vi "NSES2_Main.vi"() -> ()   [LabVIEW 2016]
uses:
  Type-Defs/Workspace.ctl
  litho folder/Global/Lithography Data.vi
panel:
  out "Workspace":T1
  in  "s_Path":path=path "C:/Users/monke/Desktop" caption="Path"
  in  "b_lithography_Monitor":bool caption="Blank"
  in  "DAQ Channel":tag
  out "Scan":picture
  out "s_InkScape_path":string="C:\\Users\\monke\\Desktop\\5.8.2018\\5.8.2018\\InkscapeFiles\\5.8.2018.000000.svg" caption="String"
  in  "b_Open_Lithography":bool caption="Config"
  in  "b_Start_Lithography":bool caption="Start"
  in  "b_Change_litho":bool caption="Change"
  in  "l_Litho_modes":i32(ring)=1 caption="Tip Signal Mode" items=["Current Measurement ", "Voltage Source", "Direct from BNC"]
  in  "b_retry_access":bool caption="Reset"
  in  "b_Lithography_Mode":bool caption="Blank"
  in  "b_Open_InkScape":bool caption="Open"
  in  "b_Save_Scan":bool caption="Save"
  in  "b_Config":bool caption="Config"
  # "InkScape should open momentarily.\nHowever, if it fails to load in a reasonable amount of time, below is the path of the InkScape file if needed:"
  # "It appears that you have not \"viewed\" the Access Codes. Please \"view\" them and then press \"RESET\"."
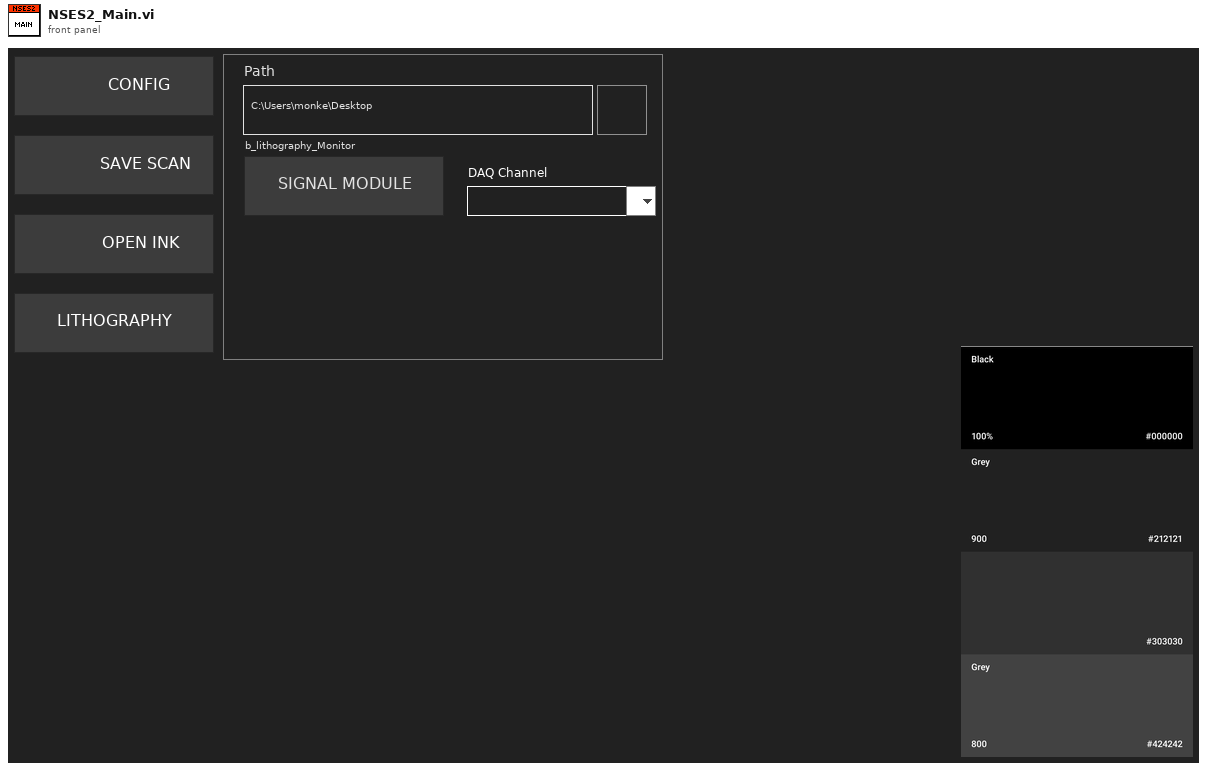
[diagram p1: front panel]
types:
  T1 = typedef "Workspace.ctl" = enum32{"CONFIG", "SAVE SCAN", "OPEN INKSCAPE", "LITHOMODE", "ERROR 97", "MONITOR_LITHO"}
  T2 = enum32{"invalid app kind", "Development System", "Run Time System", "Student Edition", "Embedded LabVIEW", "Evaluation", "Custom"}
  T3 = enum32{"Invalid", "Standard", "Closed", "Hidden", "Minimized", "Maximized"}
  T4 = cluster{"Core":cluster{"Current VI Reference":refnum<vi>, "Close Panel on Exit?":bool}, "lithography_monitor":bool, "Your string data":string, "Main_Path":path, "Image_Paths":cluster{"BMP":string, "BMP_Inkscape":string, "SVG_Inkscape":string}, "Application":refnum<k7>, "lithography_Offsets":cluster{"X":dbl, "Y":dbl}, "Lithography Data":cluster{"Name":string, "Litho":cluster{"X":dbl, "Y":dbl, "Speed":dbl, "Voltage":dbl}[]}[]}
  T5 = cluster{"Name":string, "Litho":cluster{"X":dbl, "Y":dbl, "Speed":dbl, "Voltage":dbl}[]}[]
  T6 = cluster{"BMP":string, "BMP_Inkscape":string, "SVG_Inkscape":string}
  T7 = cluster{"Current VI Reference":refnum<vi>, "Close Panel on Exit?":bool}
  T8 = enum8{"Enabled", "Disabled", "Disabled and Grayed Out"}
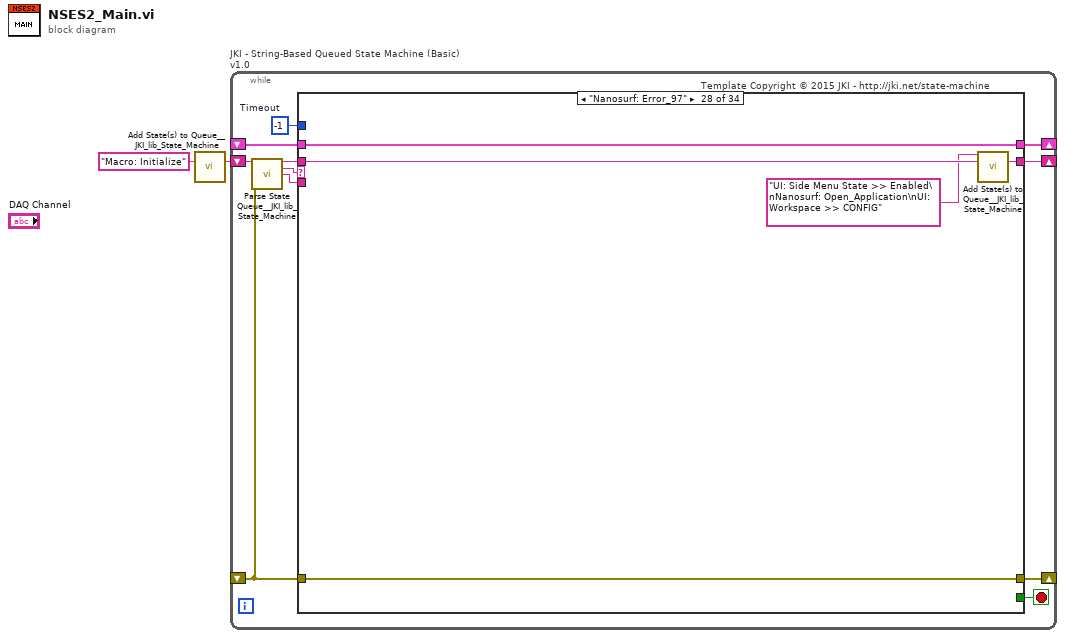
[diagram p0: block diagram]
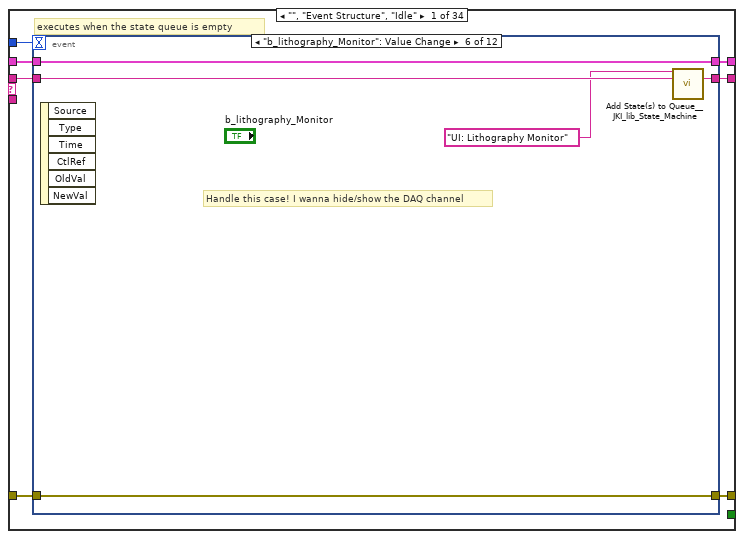
[diagram p2: hidden frame]
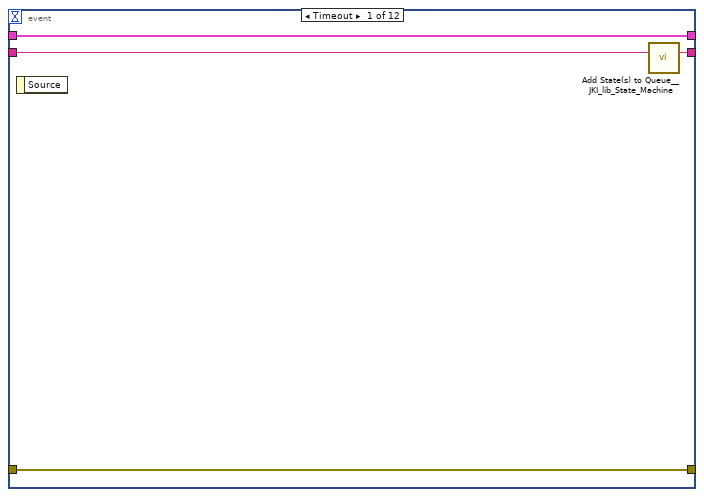
[diagram p3: hidden frame]
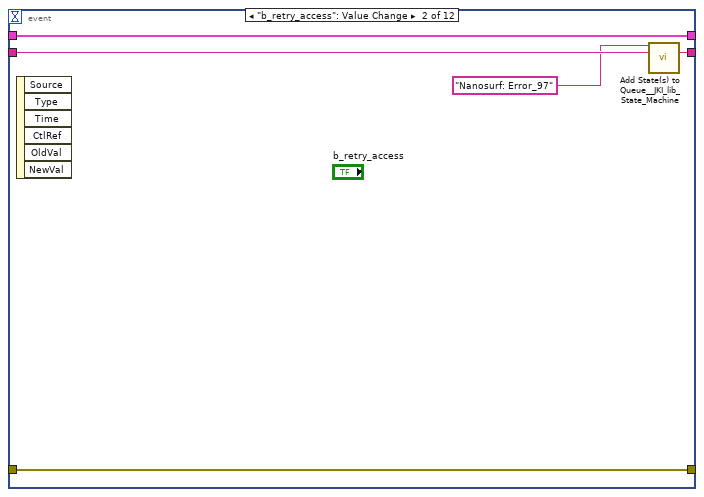
[diagram p4: hidden frame]
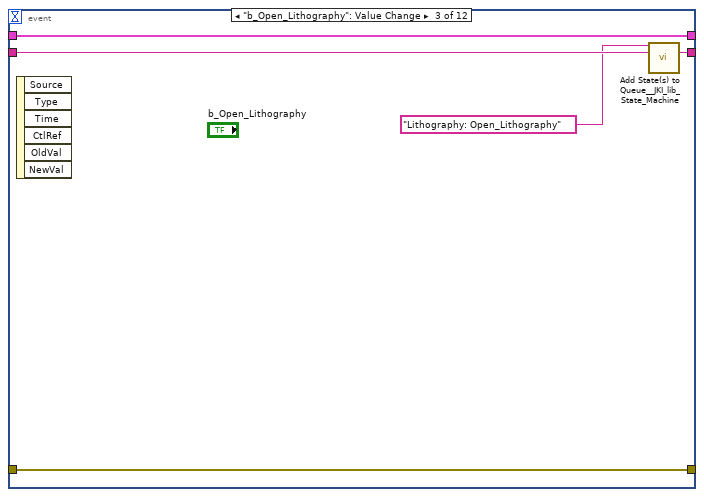
[diagram p5: hidden frame]
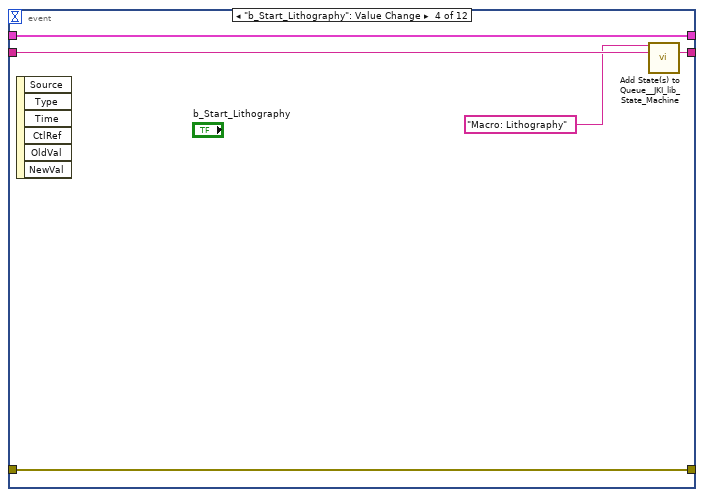
[diagram p6: hidden frame]
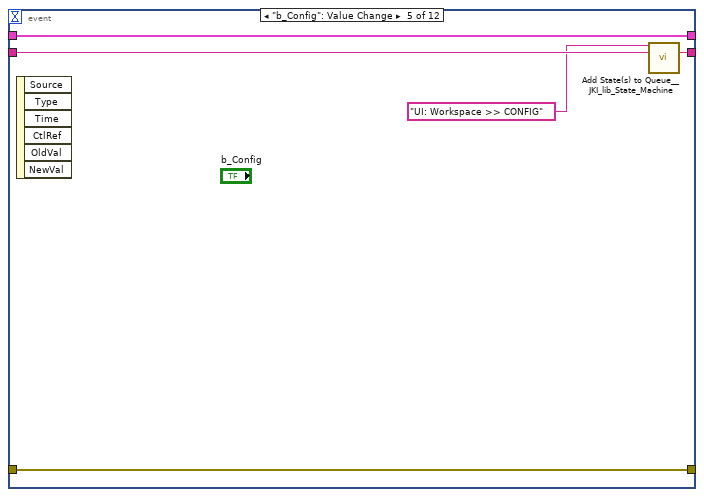
[diagram p7: hidden frame]
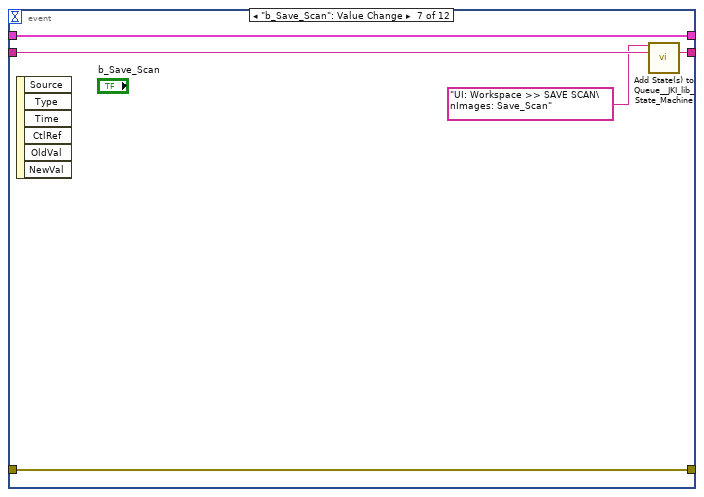
[diagram p8: hidden frame]
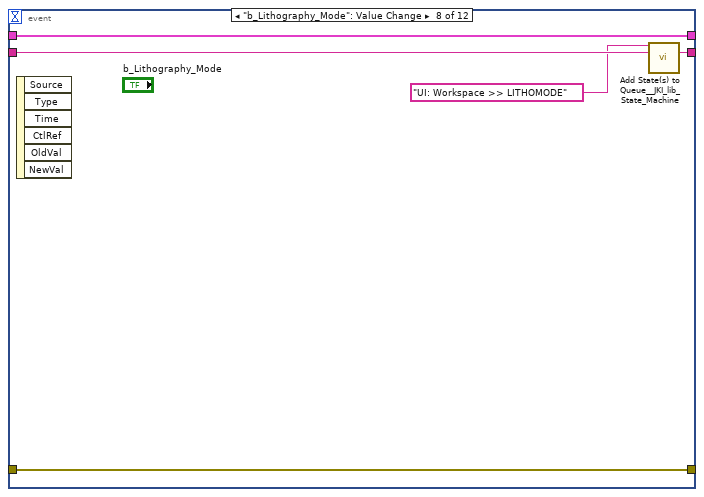
[diagram p9: hidden frame]
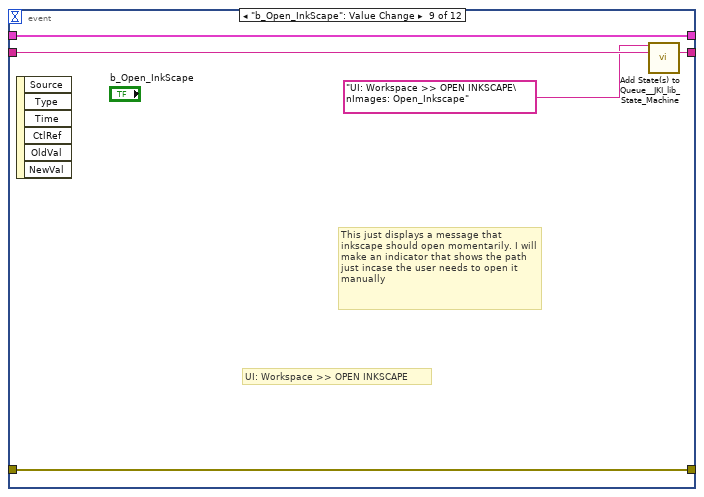
[diagram p10: hidden frame]
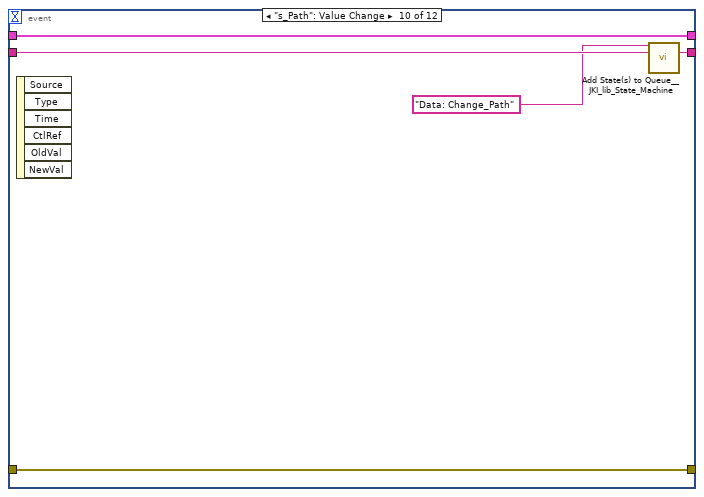
[diagram p11: hidden frame]
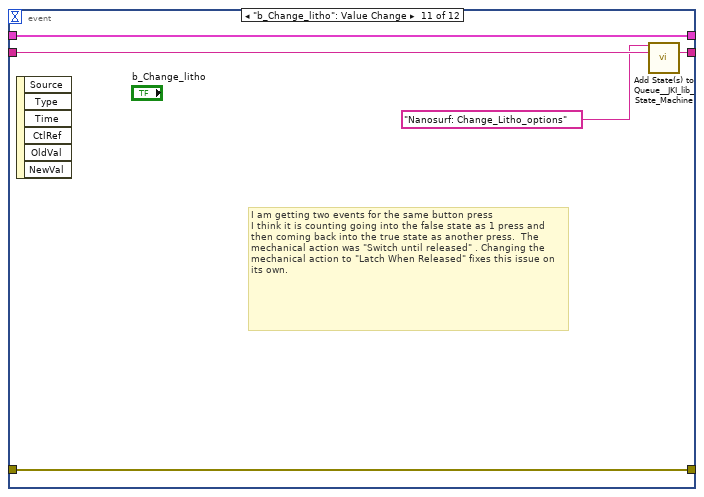
[diagram p12: hidden frame]
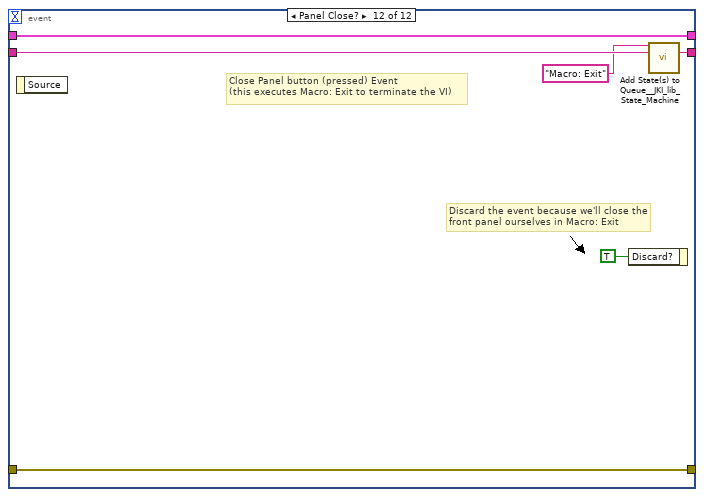
[diagram p13: hidden frame]
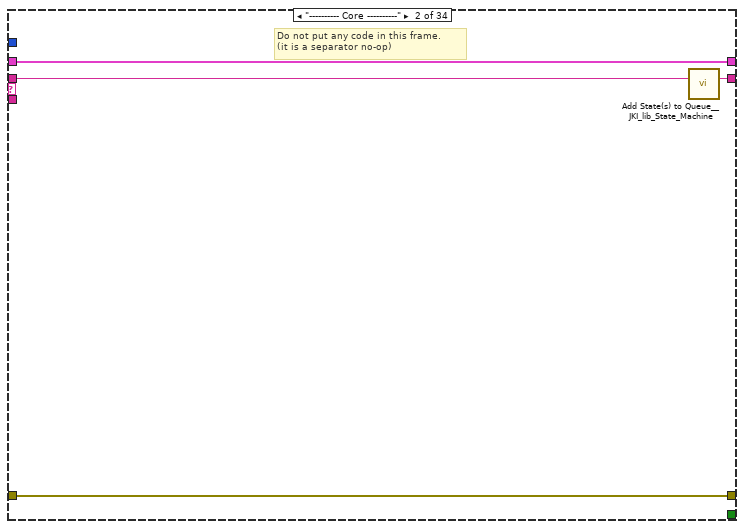
[diagram p14: hidden frame]
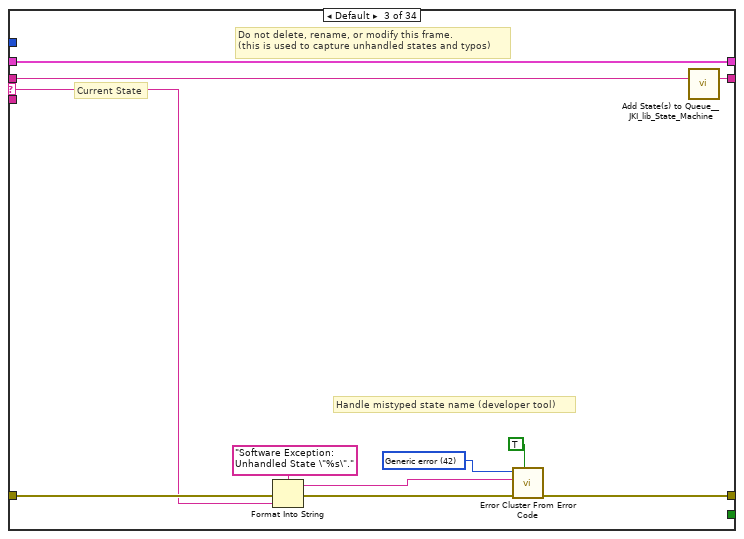
[diagram p15: hidden frame]
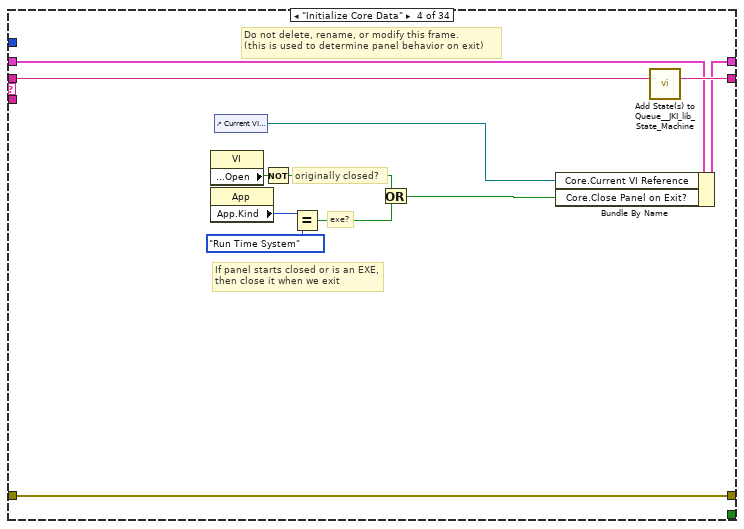
[diagram p16: hidden frame]
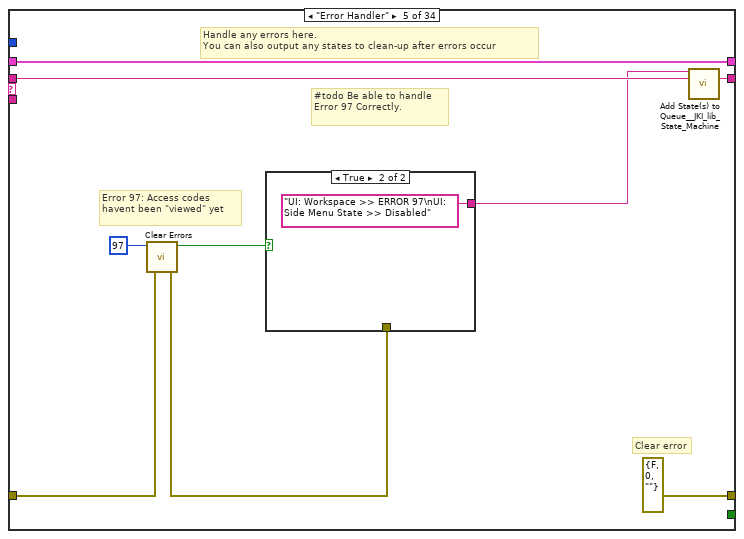
[diagram p17: hidden frame]
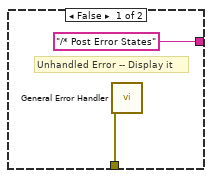
[diagram p18: hidden frame]
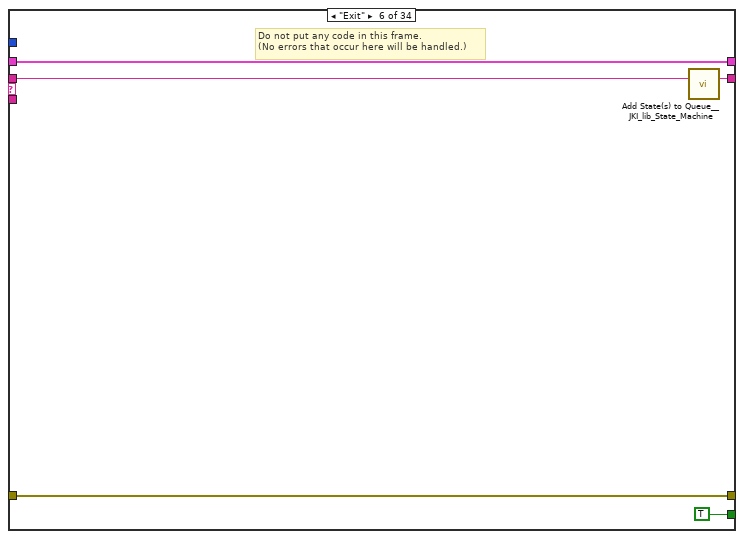
[diagram p19: hidden frame]
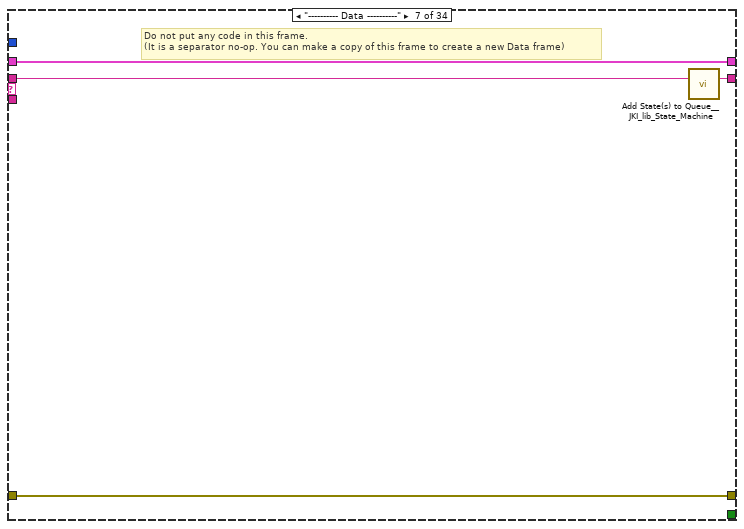
[diagram p20: hidden frame]
diagram:
  n1 = call <vilib>:"Add State(s) to Queue__JKI_lib_State_Machine.vi"("State(s) in (\"\")"="Macro: Initialize") -> ("States Out"=w2:string)  [unwired: 14 in]
  n2 = while "JKI - String-Based Queued State Machine (Basic) v1.0" {
    shift-right: [w7] -> _
    shift-left: _ -> [w6]
    shift-right: [w9] -> _
    shift-left: _ -> [w4]
    shift-right: [w3] -> _
    shift-left: w2 -> [w10]
    stop <- w8 stop-if-true
    w5 = -1  # Timeout
    # "Template Copyright © 2015 JKI - http://jki.net/state-machine"
    n3 = call <vilib>:"Parse State Queue__JKI_lib_State_Machine.vi"("State Queue"=w10, "Error In (no error)"=w4) -> ("Remaining States"=w12:string, "Current State"=w13:string, "Arguments"=w11:string)  [unwired: 11 in]
    n4 = case shown="\"Nanosurf: Error_97\"" w13 {
      selector: w13 -> [_ _ w85 _ _ _ _ _ _ _ _ _ _ _ _ _ _ _ _ _ _ _ _ _ _ _ _ _ _ _ _ _ _ _]
      tunnel: w12 -> [w20 w84 w89 w107 w116 w124 w128 w140 w146 w152 w156 w160 w166 w177 w205 w216 w234 w238 w243 w255 w265 w269 w282 w293 w297 w305 w312 w317 w323 w327 w338 w350 w359 w364]
      tunnel: w11 -> [_ _ _ _ _ _ _ _ _ _ _ _ w161 w171 w201 w211 _ _ _ _ _ _ _ _ _ _ _ _ _ _ _ _ _ w360]
      tunnel: w6 -> [w18 w81 w87 w98 w113 w122 w125 _ w143 w147 w153 w158 w164 w173 w202 w214 w230 w235 w240 w249 w262 w267 w275 w284 w294 w299 w310 w315 w319 w324 w329 w346 w355 w361]
      tunnel: [w17 w82 w91 w104 errorcluster {"status"=FALSE, "code"=0, "source"=""} ("error out") w121 w126 w137 w144 w148 w154 w157 w162 w174 w203 w212 w232 w236 w241 w253 w263 w266 w278 w285 w295 w301 w306 w313 w320 w325 w330 w340 w356 w362] -> w9
      tunnel: w4 -> [w16 w82 w90 w104 w110 w121 w126 w137 w144 w149 w154 w157 w163 w175 w203 w213 w232 w236 w241 w253 w263 w266 w279 w286 w295 w302 w307 w313 w321 w325 w331 w348 w357 w362]
      tunnel: [w19 w83 w88 w106 w115 w123 w127 w139 w145 w151 w155 w159 w165 w176 w204 w215 w233 w237 w242 w254 w264 w268 w281 w292 w296 w304 w311 w316 w322 w326 w337 w349 w358 w363] -> w3
      tunnel: [_ _ _ _ _ TRUE _ _ _ _ _ _ _ _ _ _ _ _ _ _ _ _ _ _ _ _ _ _ _ _ _ _ _ _] -> w8
      tunnel: [w15 w81 w87 w105 w113 w122 w125 w138 w142 w147 w153 w158 w164 w173 w202 w214 w229 w235 w240 w249 w262 w267 w274 w284 w294 w298 w310 w315 w319 w324 w329 w345 w355 w361] -> w7
      tunnel: w5 -> [w14 _ _ _ _ _ _ _ _ _ _ _ _ _ _ _ _ _ _ _ _ _ _ _ _ _ _ _ _ _ _ _ _ _]
      frame "", "Event Structure", "Idle" {
        # "executes when the state queue is empty"
        n5 = event shown="[5] \"b_lithography_Monitor\": Value Change" {
          selector: _ -> [_ _ _ _ _ _ _ _ _ _ _ _]
          dyn-events: _ -> [_ _ _ _ _ _ _ _ _ _ _ _]
          timeout: w14 -> [_ _ _ _ _ _ _ _ _ _ _ _]
          tunnel: w20 -> [w24 w29 w34 w39 w44 w49 w54 w59 w64 w69 w74 w80]
          tunnel: [w23 w28 w33 w38 w43 w48 w53 w58 w63 w68 w73 w79] -> w19
          tunnel: w18 -> [w21 w26 w31 w36 w41 w46 w51 w56 w61 w66 w71 w77]
          tunnel: [w22 w27 w32 w37 w42 w47 w52 w57 w62 w67 w72 w78] -> w17
          tunnel: w16 -> [w22 w27 w32 w37 w42 w47 w52 w57 w62 w67 w72 w78]
          tunnel: [w21 w26 w31 w36 w41 w46 w51 w56 w61 w66 w71 w77] -> w15
          event Timeout {
            n6 = event-data() -> ()  [unwired: 1 in, 1 out]
            n7 = call <vilib>:"Add State(s) to Queue__JKI_lib_State_Machine.vi"("State(s) in (\"\")"=w24) -> ("States Out"=w23:string)  [unwired: 14 in]
          }
          event "b_retry_access": Value Change {
            n8 = event-data() -> ()  [unwired: 1 in, 6 out]
            n9 = call <vilib>:"Add State(s) to Queue__JKI_lib_State_Machine.vi"("State(s) in Front (\"\")"="Nanosurf: Error_97" ("State(s) in Front (\"\")"), "State(s) in (\"\")"=w29) -> ("States Out"=w28:string)  [unwired: 13 in]
          }
          event "b_Open_Lithography": Value Change {
            n10 = event-data() -> ()  [unwired: 1 in, 6 out]
            n11 = call <vilib>:"Add State(s) to Queue__JKI_lib_State_Machine.vi"("State(s) in Front (\"\")"="Lithography: Open_Lithography" ("State(s) in Front (\"\")"), "State(s) in (\"\")"=w34) -> ("States Out"=w33:string)  [unwired: 13 in]
          }
          event "b_Start_Lithography": Value Change {
            n12 = event-data() -> ()  [unwired: 1 in, 6 out]
            n13 = call <vilib>:"Add State(s) to Queue__JKI_lib_State_Machine.vi"("State(s) in Front (\"\")"="Macro: Lithography" ("State(s) in Front (\"\")"), "State(s) in (\"\")"=w39) -> ("States Out"=w38:string)  [unwired: 13 in]
          }
          event "b_Config": Value Change {
            n14 = event-data() -> ()  [unwired: 1 in, 6 out]
            n15 = call <vilib>:"Add State(s) to Queue__JKI_lib_State_Machine.vi"("State(s) in Front (\"\")"="UI: Workspace >> CONFIG" ("State(s) in Front (\"\")"), "State(s) in (\"\")"=w44) -> ("States Out"=w43:string)  [unwired: 13 in]
          }
          event "b_lithography_Monitor": Value Change {
            # "Handle this case! I wanna hide/show the DAQ channel"
            n16 = event-data() -> ()  [unwired: 1 in, 6 out]
            n17 = call <vilib>:"Add State(s) to Queue__JKI_lib_State_Machine.vi"("State(s) in Front (\"\")"="UI: Lithography Monitor" ("State(s) in Front (\"\")"), "State(s) in (\"\")"=w49) -> ("States Out"=w48:string)  [unwired: 13 in]
          }
          event "b_Save_Scan": Value Change {
            n18 = event-data() -> ()  [unwired: 1 in, 6 out]
            n19 = call <vilib>:"Add State(s) to Queue__JKI_lib_State_Machine.vi"("State(s) in Front (\"\")"="UI: Workspace >> SAVE SCAN\nImages: Save_Scan" ("State(s) in Front (\"\")"), "State(s) in (\"\")"=w54) -> ("States Out"=w53:string)  [unwired: 13 in]
          }
          event "b_Lithography_Mode": Value Change {
            n20 = event-data() -> ()  [unwired: 1 in, 6 out]
            n21 = call <vilib>:"Add State(s) to Queue__JKI_lib_State_Machine.vi"("State(s) in Front (\"\")"="UI: Workspace >> LITHOMODE" ("State(s) in Front (\"\")"), "State(s) in (\"\")"=w59) -> ("States Out"=w58:string)  [unwired: 13 in]
          }
          event "b_Open_InkScape": Value Change {
            # "This just displays a message that inkscape should open momentarily. I will make an indicator that shows the path just incase the user needs to open it manually"
            # "UI: Workspace >> OPEN INKSCAPE"
            n22 = event-data() -> ()  [unwired: 1 in, 6 out]
            n23 = call <vilib>:"Add State(s) to Queue__JKI_lib_State_Machine.vi"("State(s) in Front (\"\")"="UI: Workspace >> OPEN INKSCAPE\nImages: Open_Inkscape" ("State(s) in Front (\"\")"), "State(s) in (\"\")"=w64) -> ("States Out"=w63:string)  [unwired: 13 in]
          }
          event "s_Path": Value Change {
            n24 = event-data() -> ()  [unwired: 1 in, 6 out]
            n25 = call <vilib>:"Add State(s) to Queue__JKI_lib_State_Machine.vi"("State(s) in Front (\"\")"="Data: Change_Path" ("State(s) in Front (\"\")"), "State(s) in (\"\")"=w69) -> ("States Out"=w68:string)  [unwired: 13 in]
          }
          event "b_Change_litho": Value Change {
            # "I am getting two events for the same button press \nI think it is counting going into the false state as 1 press and then coming back into the true state as another press.  The mechanical action was \"Switch until released\" . Changing the mechanical action to \"Latch When Released\" fixes this issue on its own."
            n26 = event-data() -> ()  [unwired: 1 in, 6 out]
            n27 = call <vilib>:"Add State(s) to Queue__JKI_lib_State_Machine.vi"("State(s) in Front (\"\")"="Nanosurf: Change_Litho_options", "State(s) in (\"\")"=w74) -> ("States Out"=w73:string)  [unwired: 13 in]
          }
          event Panel Close? {
            # "Discard the event because we'll close the front panel ourselves in Macro: Exit"
            # "Close Panel button (pressed) Event\n(this executes Macro: Exit to terminate the VI)"
            n28 = event-data() -> ()  [unwired: 1 in, 1 out]
            n29 = event-data("Discard?"=TRUE) -> ()  [unwired: 1 in, 1 out]
            n30 = call <vilib>:"Add State(s) to Queue__JKI_lib_State_Machine.vi"("State(s) in Front (\"\")"="Macro: Exit", "State(s) in (\"\")"=w80) -> ("States Out"=w79:string)  [unwired: 13 in]
          }
        }
      }
      frame "---------- Core ----------" {
        # "Do not put any code in this frame.\n(it is a separator no-op)"
        n31 = call <vilib>:"Add State(s) to Queue__JKI_lib_State_Machine.vi"("State(s) in (\"\")"=w84) -> ("States Out"=w83:string)  [unwired: 14 in]
      }
      frame Default {
        w94 = 42 items=["No error", "Argument error", "Memory is full", "Out of zone", "End of file", "File already open", "Generic file I/O error", "File not found", "File permission error", "Disk is full", "Duplicate path", "Too many files open", "System feature not enabled", "Resource file not found", "Cannot add resource", "Resource not found", "Image not found", "Image memory error", "Pen does not exist", "Config type invalid", "Config token not found", "Config parse error", "Config memory error", "Bad external code format", "Bad external code offset", "External code not present", "Null window", "Destroy window error", "Null menu", "Print aborted", "Bad print record", "Print driver error", "Windows error during printing", "Memory error during printing", "Print dialog error", "Generic print error", "Invalid device refnum", "Device not found", "Device parameter error", "Device unit error", "Cannot open device", "Device call aborted", "Generic error", "Cancelled by user", "Object ID too low", "Object ID too high", "Object not in heap", "Unknown heap", "Unknown object (invalid DefProc)", "Unknown object (DefProc not in table)", "Message out of range", "Invalid (null) method", "Unknown message", "Manager call not supported", "Bad address", "Network operation in progress", "Network operation timed out", "Connection is busy", "Network attribute not supported", "Network error", "Address in use", "System out of memory", "Connection aborted", "Connection refused", "Not connected", "Already connected", "Connection closed", "Initialization error (interapplication manager)", "Bad occurrence", "Wait on unbound occurrence handler", "Occurrence queue overflow", "Datalog type conflict", "Unused", "Unrecognized type (interapplication manager)", "Memory corrupt", "Failed to make temporary DLL", "Old CIN version", "Drag socket not found", "Failed to load drop-object", "Failed to register OLE object", "Failed to release OLE object", "Format specifier type mismatch", "Unknown format specifier", "Too few format specifiers", "Too many format specifiers", "Scan failed", "Newer CIN version", "Error converting to variant", "Runtime menu error", "Password tampered", "Variant attribute not found", "Incompatible variant data type", "Event data is not available", "Event Store is not present", "Occurrence is not found", "Event Queue is not created", "Event info is not available", "Refnum passed is NULL", "Error retrieving Class GUID", "Error retrieving CoClass GUID", "Error retrieving TypeLib GUID.", "Bad built application magic bytes.", "Specific driver is different from the specific driver associated with the Logical Name.", "There is no session opened to the class driver.", "Max Error", "MAX - Error with config objects", "MAX - Error loading configuration", "MAX - Group not supported"]
        # "Current State"
        # "Do not delete, rename, or modify this frame.\n(this is used to capture unhandled states and typos)"
        # "Handle mistyped state name (developer tool)"
        n32 = Format Into String(format string="Software Exception: Unhandled State \"%s\"." ("message"), error in=w90, w85) -> (resulting string=w93:string, error out=w92:errorcluster)  [unwired: 1 in]
        n33 = call <vilib>:"Error Cluster From Error Code.vi"("show call chain? (False)"=TRUE, "error in (no error)"=w92, "error message (\"\")"=w93, "error code (0)"=w94) -> ("error out"=w91:errorcluster)  [unwired: 5 in]
        n34 = call <vilib>:"Add State(s) to Queue__JKI_lib_State_Machine.vi"("State(s) in (\"\")"=w89) -> ("States Out"=w88:string)  [unwired: 14 in]
      }
      frame "Initialize Core Data" {
        # "Do not delete, rename, or modify this frame.\n(this is used to determine panel behavior on exit)"
        # "originally closed?"
        # "exe?"
        # "If panel starts closed or is an EXE, then close it when we exit"
        n35 = property class="VI"() -> ("Front Panel.Open"=w103:bool)  [unwired: 2 in, 2 out]
        n36 = property class="App"() -> ("App.Kind"=w102:T2)  [unwired: 2 in, 2 out]
        n37 = control-ref of="Current VI Reference"() -> (w96:refnum<vi>)
        n38 = Not(x=w103) -> (.not. x?=w100:bool)
        n39 = Equal?(x=w102, y=T2."Run Time System" ("Application:Kind")) -> (x = y?=w99:bool)
        n40 = Or(x=w100, y=w99) -> (x .or. y?=w97:bool)
        n41 = Bundle By Name(cluster=w98, "Core.Current VI Reference"=w96, "Core.Close Panel on Exit?"=w97) -> (w105:T4)
        n42 = call <vilib>:"Add State(s) to Queue__JKI_lib_State_Machine.vi"("State(s) in (\"\")"=w107) -> ("States Out"=w106:string)  [unwired: 14 in]
      }
      frame "Error Handler" {
        # "Error 97: Access codes havent been \"viewed\" yet"
        # "#todo Be able to handle Error 97 Correctly."
        # "Handle any errors here.\nYou can also output any states to clean-up after errors occur"
        # "Clear error"
        n43 = call <vilib>:"Clear Errors.vi"("error in (no error)"=w110, "specific error code to clear (0: all)"=97) -> ("error out"=w109:errorcluster, "specific error cleared?"=w111:bool)  [unwired: 4 in]
        n44 = case shown="True" w111 {
          tunnel: w109 -> [w118 _]
          tunnel: ["/* Post Error States" "UI: Workspace >> ERROR 97\nUI: Side Menu State >> Disabled"] -> w108
          frame False {
            # "Unhandled Error -- Display it"
            n45 = call <vilib>:"General Error Handler.vi"("error in (no error)"=w118) -> ()  [unwired: 10 in, 5 out]
          }
          frame True {
          }
        }
        n46 = call <vilib>:"Add State(s) to Queue__JKI_lib_State_Machine.vi"("State(s) in Front (\"\")"=w108, "State(s) in (\"\")"=w116) -> ("States Out"=w115:string)  [unwired: 13 in]
      }
      frame "Exit" {
        # "Do not put any code in this frame.\n(No errors that occur here will be handled.)"
        n47 = call <vilib>:"Add State(s) to Queue__JKI_lib_State_Machine.vi"("State(s) in (\"\")"=w124) -> ("States Out"=w123:string)  [unwired: 14 in]
      }
      frame "---------- Data ----------" {
        # "Do not put any code in this frame.\n(It is a separator no-op. You can make a copy of this frame to create a new Data frame)"
        n48 = call <vilib>:"Add State(s) to Queue__JKI_lib_State_Machine.vi"("State(s) in (\"\")"=w128) -> ("States Out"=w127:string)  [unwired: 14 in]
      }
      frame "Data: Initialize" {
        w129 = T5 []  # Lithography Data
        w130 = cluster{"X":dbl, "Y":dbl} {"X"=0.0, "Y"=0.0}  # lithography_Offsets
        w131 = refnum<k7> refnum  # Application
        w132 = T6 {"BMP"="", "BMP_Inkscape"="", "SVG_Inkscape"=""}  # Image_Paths
        w133 = path ""  # Main_Path
        w134 = T7 {"Current VI Reference"=refnum, "Close Panel on Exit?"=FALSE}  # Core
        w136 = TRUE  # lithography_monitor
        w135 = ""  # Your string data
        # "Initialize the shift-register data, here.\n(data names are defined by what you wire into the bundle function)"
        n49 = Bundle("Core"=w134, "lithography_monitor"=w136, "Your string data"=w135, "Main_Path"=w133, "Image_Paths"=w132, "Application"=w131, "lithography_Offsets"=w130, "Lithography Data"=w129) -> (w138:T4)  [unwired: 1 in]
        n50 = call <vilib>:"Add State(s) to Queue__JKI_lib_State_Machine.vi"("State(s) in (\"\")"=w140) -> ("States Out"=w139:string)  [unwired: 14 in]
      }
      frame "Data: Change_Path" {
        # "Do not put any code in this frame.\n(It is a separator no-op. You can make a copy of this frame to create a new Data frame)"
        n51 = Bundle By Name(cluster=w143, "Main_Path"="s_Path") -> (w142:T4)
        n52 = call <vilib>:"Add State(s) to Queue__JKI_lib_State_Machine.vi"("State(s) in (\"\")"=w146) -> ("States Out"=w145:string)  [unwired: 14 in]
      }
      frame "Data: Cleanup" {
        # "Cleanup any data and references, here.\n(this is called automatically, by the Macro: Exit)"
        n53 = Unbundle By Name(w147) -> ("Core.Current VI Reference"=w150:refnum<vi>)
        n54 = Close Reference(reference=w150, error in (no error)=w149) -> (error out=w148:errorcluster)
        n55 = call <vilib>:"Add State(s) to Queue__JKI_lib_State_Machine.vi"("State(s) in (\"\")"=w152) -> ("States Out"=w151:string)  [unwired: 14 in]
      }
      frame "---------- UI ----------" {
        # "Do not put any code in this frame.\n(It is a separator no-op. You can make a copy of this frame to create a new UI frame)"
        n56 = call <vilib>:"Add State(s) to Queue__JKI_lib_State_Machine.vi"("State(s) in (\"\")"=w156) -> ("States Out"=w155:string)  [unwired: 14 in]
      }
      frame "UI: Initialize" {
        # "Initialize the User Interface, here.\n(this is called automatically, by the Macro: Init)"
        n57 = call <vilib>:"Add State(s) to Queue__JKI_lib_State_Machine.vi"("State(s) in (\"\")"=w160) -> ("States Out"=w159:string)  [unwired: 14 in]
      }
      frame "UI: Cursor Set" {
        # "Argument"
        # "Set and Unset Cursor Busy.\n(Usage: \"UI: Cursor Set >> Busy|Idle\")"
        n58 = case shown="\"Idle\", Default" w161 {
          tunnel: w163 -> [w168 w170]
          tunnel: [w167 w169] -> w162
          frame "Idle", Default {
            n59 = call <vilib>:"Unset Busy.vi"("error in (no error)"=w168) -> ("error out"=w167:errorcluster)  [unwired: 10 in]
          }
          frame "Busy" {
            n60 = call <vilib>:"Set Busy.vi"("error in (no error)"=w170) -> ("error out"=w169:errorcluster)  [unwired: 9 in, 1 out]
          }
        }
        n61 = call <vilib>:"Add State(s) to Queue__JKI_lib_State_Machine.vi"("State(s) in (\"\")"=w166) -> ("States Out"=w165:string)  [unwired: 14 in]
      }
      frame "UI: Front Panel State" {
        # "Argument"
        # "Set Front Panel Open or Closed\n(Usage: \"UI: Front Panel State >> Open|Close\")"
        n62 = Unbundle By Name(w173) -> ("Core.Current VI Reference"=w172:refnum<vi>)
        n63 = case shown="\"Open\", Default" w171 {
          tunnel: w175 -> [w181 w194]
          tunnel: [w183 w195] -> w174
          tunnel: w172 -> [w182 w192]
          frame "Open", Default {
            n64 = property class="VI"(reference=w182, error in=w181) -> (reference out=w179:refnum<vi>, error out=w180:errorcluster, "Front Panel.Open"=w178:bool)
            n65 = case shown="False" w178 {
              tunnel: [w186 w189] -> w183
              tunnel: w180 -> [w185 w189]
              tunnel: w179 -> [w184 _]
              frame False {
                n66 = invoke class="VI" method="FP.Open"(reference=w184, error in=w185, "Activate"=TRUE, "State"=T3."Standard") -> (error out=w186:errorcluster)  [unwired: 1 in, 4 out]
              }
              frame True {
              }
            }
          }
          frame "Close" {
            n67 = property class="VI"(reference=w192, error in=w194) -> (reference out=w191:refnum<vi>, error out=w193:errorcluster, "Front Panel.Open"=w190:bool)
            n68 = case shown="True" w190 {
              tunnel: [w196 w199] -> w195
              tunnel: w193 -> [w196 w198]
              tunnel: w191 -> [_ w197]
              frame False {
              }
              frame True {
                n69 = invoke class="VI" method="FP.Close"(reference=w197, error in=w198) -> (error out=w199:errorcluster)  [unwired: 1 in, 2 out]
              }
            }
          }
        }
        n70 = call <vilib>:"Add State(s) to Queue__JKI_lib_State_Machine.vi"("State(s) in (\"\")"=w177) -> ("States Out"=w176:string)  [unwired: 14 in]
      }
      frame "UI: Workspace" {
        # "Workspace Tab State\n(This is the frame that changes the Workspace Value)"
        n71 = case shown="\"CONFIG\", Default" w201 {
          tunnel: [Workspace."CONFIG" ("Workspace") Workspace."SAVE SCAN" ("Workspace") Workspace."OPEN INKSCAPE" ("Workspace") Workspace."ERROR 97" ("Workspace") Workspace."LITHOMODE" ("Workspace")] -> w200
          frame "CONFIG", Default {
            # "UI: Workspace >> CONFIG"
          }
          frame "SAVE SCAN" {
            # "UI: Workspace >> SAVE SCAN"
          }
          frame "OPEN INKSCAPE" {
            # "UI: Workspace >> OPEN INKSCAPE"
          }
          frame "ERROR 97" {
            # "UI: Workspace >> ERROR 97"
          }
          frame "LITHOMODE" {
            # "UI: Workspace >> LITHOMODE"
          }
        }
        "Workspace" <- w200
        n72 = call <vilib>:"Add State(s) to Queue__JKI_lib_State_Machine.vi"("State(s) in (\"\")"=w205) -> ("States Out"=w204:string)  [unwired: 14 in]
      }
      frame "UI: Side Menu State" {
        # "Do not put any code in this frame.\n(It is a separator no-op. You can make a copy of this frame to create a new UI frame)"
        n73 = case shown="\"Disabled\"" w211 {
          tunnel: w213 -> [w222 w228]
          tunnel: [w221 w227] -> w212
          frame "Disabled" {
            w217 = T8."Disabled and Grayed Out" ("Disabled")
            n74 = property on="b_Config" class="Bool"(error in=w222, "DisabledEnum"=w217) -> (error out=w218:errorcluster)  [unwired: 1 in, 1 out]
            n75 = property on="b_Save_Scan" class="Bool"(error in=w218, "DisabledEnum"=w217) -> (error out=w219:errorcluster)  [unwired: 1 in, 1 out]
            n76 = property on="b_Open_InkScape" class="Bool"(error in=w219, "DisabledEnum"=w217) -> (error out=w220:errorcluster)  [unwired: 1 in, 1 out]
            n77 = property on="b_Lithography_Mode" class="Bool"(error in=w220, "DisabledEnum"=w217) -> (error out=w221:errorcluster)  [unwired: 1 in, 1 out]
          }
          frame "Enabled", Default {
            w223 = T8."Enabled" ("Disabled")
            n78 = property on="b_Config" class="Bool"(error in=w228, "DisabledEnum"=w223) -> (error out=w224:errorcluster)  [unwired: 1 in, 1 out]
            n79 = property on="b_Save_Scan" class="Bool"(error in=w224, "DisabledEnum"=w223) -> (error out=w225:errorcluster)  [unwired: 1 in, 1 out]
            n80 = property on="b_Open_InkScape" class="Bool"(error in=w225, "DisabledEnum"=w223) -> (error out=w226:errorcluster)  [unwired: 1 in, 1 out]
            n81 = property on="b_Lithography_Mode" class="Bool"(error in=w226, "DisabledEnum"=w223) -> (error out=w227:errorcluster)  [unwired: 1 in, 1 out]
          }
        }
        n82 = call <vilib>:"Add State(s) to Queue__JKI_lib_State_Machine.vi"("State(s) in (\"\")"=w216) -> ("States Out"=w215:string)  [unwired: 14 in]
      }
      frame "UI: Lithography Monitor" {
        # "#b_lithography_Monitor"
        # "Do not put any code in this frame.\n(It is a separator no-op. You can make a copy of this frame to create a new UI frame)"
        n83 = local read "b_lithography_Monitor"() -> (w231:bool)
        n84 = Bundle By Name(cluster=w230, "lithography_monitor"=w231) -> (w229:T4)
        n85 = property on="DAQ Channel" class="DAQName"("Visible"=w231) -> ()  [unwired: 2 in, 2 out]
        n86 = call <vilib>:"Add State(s) to Queue__JKI_lib_State_Machine.vi"("State(s) in (\"\")"=w234) -> ("States Out"=w233:string)  [unwired: 14 in]
      }
      frame "---------- Macro ----------" {
        # "Do not put any code in this frame.\n(It is a separator no-op. You can make a copy of this frame to create a new Macro frame)"
        n87 = call <vilib>:"Add State(s) to Queue__JKI_lib_State_Machine.vi"("State(s) in (\"\")"=w238) -> ("States Out"=w237:string)  [unwired: 14 in]
      }
      frame "Macro: Initialize" {
        w239 = "Data: Initialize\nInitialize Core Data\nUI: Initialize\nUI: Front Panel State >> Open\nUI: Workspace >> CONFIG\nUI: Lithography Monitor\nNanosurf: Open_Application\nData: Change_Path"  # Data: Initialize Initialize Core Data UI: Initialize UI: Front Panel State >> Open UI: Workspace >> CONFIG UI: Lithography Monitor Nanosurf: Open_Application Data: Change_Path
        # "Initialization Macro\n(This is called once, when the VI starts)"
        n88 = call <vilib>:"Add State(s) to Queue__JKI_lib_State_Machine.vi"("State(s) in Front (\"\")"=w239, "State(s) in (\"\")"=w243) -> ("States Out"=w242:string)  [unwired: 13 in]
      }
      frame "Macro: Lithography" {
        # "Do not put any code in this frame.\n(It is a separator no-op. You can make a copy of this frame to create a new Macro frame)"
        n89 = Unbundle By Name(w249) -> ("lithography_monitor"=w248:bool)
        n90 = Select(t="DAQ Card" ("State"), s=w248, f="Signal Module" ("State")) -> (s? t:f=w251:string)
        n91 = call <vilib>:"Build State String with Arguments__JKI_lib_State_Machine.vi"("Arguments (\"\")"=w251, "State"="Lithography: Run") -> ("State with Arguments"=w246:string)  [unwired: 4 in]
        n92 = call <vilib>:"Add State(s) to Queue__JKI_lib_State_Machine.vi"("State(s) in (\"\")"="Lithography: Init\nLithography: Queue", "State(s) at Back (\"\")"=w246) -> ("States Out"=w244:string)  [unwired: 13 in]
        n93 = call <vilib>:"Add State(s) to Queue__JKI_lib_State_Machine.vi"("State(s) in Front (\"\")"=w244, "State(s) in (\"\")"=w255) -> ("States Out"=w254:string)  [unwired: 13 in]
      }
      frame "Macro: Exit" {
        # "Exit Macro\n(This is called once, when the VI exits)"
        n94 = Unbundle By Name(w262) -> ("Core.Close Panel on Exit?"=w261:bool)
        n95 = Select(t="UI: Front Panel State >> Close", s=w261, f="") -> (s? t:f=w258:string)
        n96 = call <vilib>:"Add State(s) to Queue__JKI_lib_State_Machine.vi"("State(s) in (\"\")"=w258, "State(s) at Back (\"\")"="UI: Workspace >> CONFIG\nNanosurf: Close_Application\nData: Cleanup\nExit") -> ("States Out"=w256:string)  [unwired: 13 in]
        n97 = call <vilib>:"Add State(s) to Queue__JKI_lib_State_Machine.vi"("State(s) in Front (\"\")"=w256, "State(s) in (\"\")"=w265) -> ("States Out"=w264:string)  [unwired: 13 in]
      }
      frame "---------- Images ----------" {
        # "Template Separator\n(You can make a copy of, or modify, this frame)"
        n98 = call <vilib>:"Add State(s) to Queue__JKI_lib_State_Machine.vi"("State(s) in (\"\")"=w269) -> ("States Out"=w268:string)  [unwired: 14 in]
      }
      frame "Images: Save_Scan" {
        # "Template Separator\n(This will make an make a copy of, or modify, this frame)"
        n99 = Unbundle By Name(w275) -> ("Application"=w270:refnum<k7>, "Main_Path"=w276:path)
        n100 = call "Generic file paths.vi"("error in (no error)"=w279, "Parent Folder"=w276) -> ("error out"=w280:errorcluster, "SVG Path"=w271:string, "BMP for inkscape path"=w272:string, "BMP Path"=w273:string)  [unwired: 6 in]
        n101 = call "Save_Scan_macro.vi"("Application"=w270, "error in (no error)"=w280, "InkScape"=w271, "BMP INK Path"=w272, "BMP Path"=w273) -> ("error out"=w278:errorcluster, "BMP"=→"Scan":picture)  [unwired: 5 in]
        n102 = Bundle By Name(cluster=w275, "Image_Paths.BMP"=w273, "Image_Paths.BMP_Inkscape"=w272, "Image_Paths.SVG_Inkscape"=w271) -> (w274:T4)
        n103 = call <vilib>:"Add State(s) to Queue__JKI_lib_State_Machine.vi"("State(s) in (\"\")"=w282) -> ("States Out"=w281:string)  [unwired: 14 in]
      }
      frame "Images: Open_Inkscape" {
        # "Template Separator\n(You can make a copy of, or modify, this frame)"
        n104 = Unbundle By Name(w284) -> ("Image_Paths.SVG_Inkscape"=w283:string)
        "s_InkScape_path" <- w283
        n105 = Concatenate Strings("cmd /c \"", w283, "\"") -> (w289:string)
        n106 = call <vilib>:"System Exec.vi"("run minimized? (F)"=TRUE, "wait until completion? (T)"=FALSE, "error in (no error)"=w286, "command line"=w289) -> ("error out"=w285:errorcluster)  [unwired: 4 in, 3 out]
        n107 = call <vilib>:"Add State(s) to Queue__JKI_lib_State_Machine.vi"("State(s) in (\"\")"=w293) -> ("States Out"=w292:string)  [unwired: 14 in]
      }
      frame "---------- Nanosurf ----------" {
        # "Template Separator\n(You can make a copy of, or modify, this frame)"
        n108 = call <vilib>:"Add State(s) to Queue__JKI_lib_State_Machine.vi"("State(s) in (\"\")"=w297) -> ("States Out"=w296:string)  [unwired: 14 in]
      }
      frame "Nanosurf: Open_Application" {
        n109 = Unbundle By Name(w299) -> ("Application"=w303:refnum<k7>)
        n110 = Automation Open(error in (no error)=w302, Automation Refnum=w303) -> (Automation Refnum=w300:refnum<k7>, error out=w301:errorcluster)  [unwired: 2 in]
        n111 = Bundle By Name(cluster=w299, "Application"=w300) -> (w298:T4)
        n112 = call <vilib>:"Add State(s) to Queue__JKI_lib_State_Machine.vi"("State(s) in (\"\")"=w305) -> ("States Out"=w304:string)  [unwired: 14 in]
      }
      frame "Nanosurf: Change_Litho_options" {
        # "Change Lithography Options\n(Changes what the microscope uses to source the tip voltage. [more options may be added later])"
        n113 = Unbundle By Name(w310) -> ("Application"=w309:refnum<k7>)
        n114 = call "Change_tip_signal.vi"("error in (no error)"=w307, "l_Litho_modes"="l_Litho_modes", "Application"=w309) -> ("error out"=w306:errorcluster)  [unwired: 8 in]
        n115 = call <vilib>:"Add State(s) to Queue__JKI_lib_State_Machine.vi"("State(s) in (\"\")"=w312) -> ("States Out"=w311:string)  [unwired: 14 in]
      }
      frame "Nanosurf: Error_97" {
        n116 = call <vilib>:"Add State(s) to Queue__JKI_lib_State_Machine.vi"("State(s) in Front (\"\")"="UI: Side Menu State >> Enabled\nNanosurf: Open_Application\nUI: Workspace >> CONFIG", "State(s) in (\"\")"=w317) -> ("States Out"=w316:string)  [unwired: 13 in]
      }
      frame "Nanosurf: Close_Application" {
        # "Template Separator\n(You can make a copy of, or modify, this frame)"
        n117 = Unbundle By Name(w319) -> ("Application"=w318:refnum<k7>)
        n118 = Close Reference(reference=w318, error in (no error)=w321) -> (error out=w320:errorcluster)
        n119 = call <vilib>:"Add State(s) to Queue__JKI_lib_State_Machine.vi"("State(s) in (\"\")"=w323) -> ("States Out"=w322:string)  [unwired: 14 in]
      }
      frame "---------- Lithography ----------" {
        # "Template Separator\n(You can make a copy of, or modify, this frame)"
        n120 = call <vilib>:"Add State(s) to Queue__JKI_lib_State_Machine.vi"("State(s) in (\"\")"=w327) -> ("States Out"=w326:string)  [unwired: 14 in]
      }
      frame "Lithography: Open_Lithography" {
        w328 = ""  # Lithography program path
        # "Template Separator\n(You can make a copy of, or modify, this frame)"
        n121 = call "Display Message to User"() -> ()  [unwired: 10 in, 2 out]
        n122 = Concatenate Strings("cmd /c \"", w328, "\"") -> (w334:string)
        n123 = call <vilib>:"System Exec.vi"("run minimized? (F)"=TRUE, "wait until completion? (T)"=FALSE, "error in (no error)"=w331, "command line"=w334) -> ("error out"=w330:errorcluster)  [unwired: 4 in, 3 out]
        n124 = call <vilib>:"Add State(s) to Queue__JKI_lib_State_Machine.vi"("State(s) in (\"\")"=w338) -> ("States Out"=w337:string)  [unwired: 14 in]
      }
      frame "Lithography: Init" {
        # "I get wierd Error handling Behavior since I have the lithography data disabled as of right now. So the for loop in change litho units never gets executed"
        # "Initialize Lithography\n(Takes care of all of the parts of the driver that can be done ahead of time)"
        n125 = disable-structure shown="Disabled" {
          disable-tunnel: [w351 _] -> w343
          frame Disabled {
            n126 = global read "Lithography Data.vi" "Lithography Data"() -> (w351:T5)
          }
          frame Enabled {
          }
        }
        n127 = Unbundle By Name(w346) -> ("Application"=w347:refnum<k7>)
        n128 = call "Initialize_Lithography.vi"("error in"=w348, "Application"=w347) -> ("error out"=w339:errorcluster, "lithography_Offsets"=w344:cluster{"X":dbl, "Y":dbl})  [unwired: 8 in]
        n129 = call "Convert to meters.vi"("error in (no error)"=w339, "Lithography Data In"=w343) -> ("error out"=w341:errorcluster, "Lithography Data Out"=w342:T5)  [unwired: 8 in]
        n130 = Merge Errors(w341, w339) -> (w340:errorcluster)
        n131 = Bundle By Name(cluster=w346, "lithography_Offsets"=w344, "Lithography Data"=w342) -> (w345:T4)
        n132 = call <vilib>:"Add State(s) to Queue__JKI_lib_State_Machine.vi"("State(s) in (\"\")"=w350) -> ("States Out"=w349:string)  [unwired: 14 in]
      }
      frame "Lithography: Queue" {
        # "Template Separator\n(You can make a copy of, or modify, this frame)"
        n133 = Unbundle By Name(w355) -> ("Application"=w354:refnum<k7>, "Lithography Data"=w353:T5, "lithography_Offsets"=w352:cluster{"X":dbl, "Y":dbl})
        n134 = call "Queue_Macro.vi"("error in"=w357, "lithography_Offsets"=w352, "Lithography Data In"=w353, "Application"=w354) -> ("error out"=w356:errorcluster)  [unwired: 7 in]
        n135 = call <vilib>:"Add State(s) to Queue__JKI_lib_State_Machine.vi"("State(s) in (\"\")"=w359) -> ("States Out"=w358:string)  [unwired: 14 in]
      }
      frame "Lithography: Run" {
        n136 = case shown="\"False\", Default" w360 {
          frame "False", Default {
            n137 = while {
              stop <- TRUE stop-if-true
            }
          }
          frame "True" {
            n138 = while {
              stop <- TRUE stop-if-true
            }
          }
        }
        n139 = call <vilib>:"Add State(s) to Queue__JKI_lib_State_Machine.vi"("State(s) in (\"\")"=w364) -> ("States Out"=w363:string)  [unwired: 14 in]
      }
    }
  }
